vi "half cos filter tester.vi"() -> ()   [LabVIEW 2021]
uses:
  <instrlib>/_niInstr/Basic Elements/v1/FPGA/niInstr Basic Elements v1 FPGA.lvlib
panel:
  out "Waveform Chart 2":dbl(graph)
  in  "Stop":bool
  out "Waveform Chart":dbl(graph)
  in  "s":bool
  in  "input valid":bool=TRUE
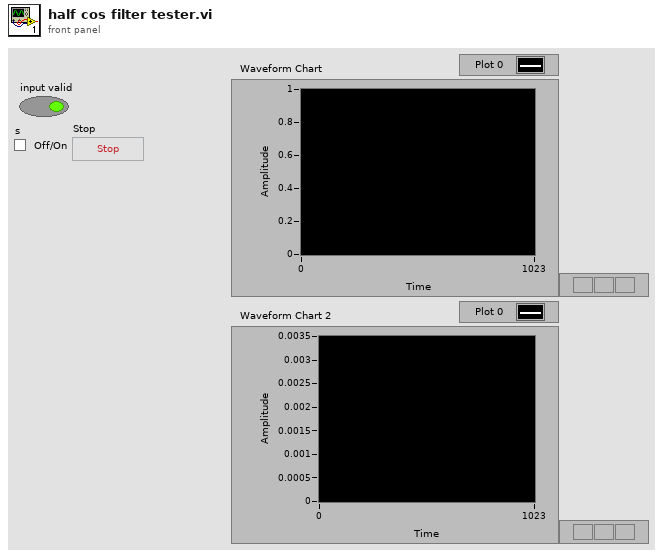
[diagram p1: front panel]
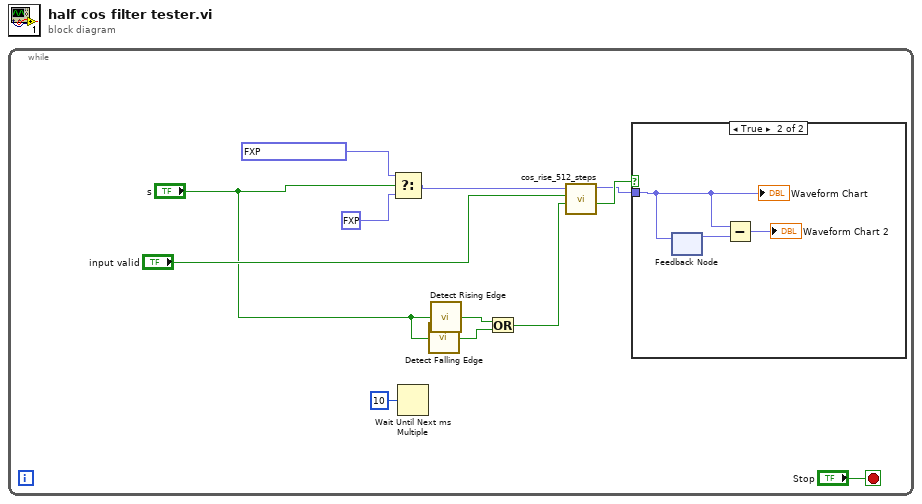
[diagram p0: block diagram]
diagram:
  n1 = while {
    stop <- "Stop" stop-if-true
    n2 = Select(t=fxp<+/-,16,1> 0.999969482421875 ("data in"), s="s", f=fxp<+/-,16,1> 0.0 ("data in")) -> (s? t:f=w11:fxp<+/-,16,1>)
    n3 = Wait Until Next ms Multiple(millisecond multiple=u32 10) -> ()  [unwired: 1 out]
    n4 = call <instrlib>:"Detect Falling Edge.vi"("signal"="s") -> ("edge detected"=w6:bool)  [unwired: 14 in]
    n5 = call <instrlib>:"Detect Rising Edge.vi"("signal"="s") -> ("edge detected"=w7:bool)  [unwired: 14 in]
    n6 = Or(x=w7, y=w6) -> (x .or. y?=w8:bool)
    n7 = call "cos_rise_512_steps.vi"("new step"=w8, "input valid"="input valid", "data in"=w11) -> ("output valid"=w4:bool, "data out"=w3:fxp<+/-,16,1>)  [unwired: 6 in, 1 out]
    n8 = case shown="True" w4 {
      tunnel: w3 -> [_ w15]
      frame False {
      }
      frame True {
        n9 = feedback-in #1(w15) -> ()
        n10 = feedback #1() -> (w14:fxp<+/-,16,1>)  [unwired: 1 in]
        n11 = Subtract(x=w15, y=w14) -> (x-y=→"Waveform Chart 2":fxp<+/-,17,2>)
        "Waveform Chart" <- w15
      }
    }
  }
